vi "Autonomous Independent.vi"   [LabVIEW 2011]
doc: "This VI is called when autonomous begins, and will automatically be terminated when autonomous ends. You can carry out timed or sensor driven robot movement independently without needing to return to the caller."
uses:
  Robot Global Data.vi
  <vilib>/Rock Robotics/WPI/RobotDrive/WPI_RobotDriveArcadeDrive_Standard(NoSaturation).vi
types:
  T1 = typedef "WPI_RobotDriveDevRef.ctl" = cluster{"DevStatus":errorcluster, "Motors[]":T2[], "Square Inputs":bool, "Max Output":dbl, "Isochronous":bool}
  T2 = typedef "WPI_MotorControlDeviceRef.ctl" = cluster{"DeviceStatus":errorcluster, "Type":enum16{"PWM", "CAN"}, "PWM":cluster{"Digital Module":T3, "PWM Channel":T4, "DeadBand":T5}, "CAN":cluster{"Device Number":u8, "Control Mode":T6, "Semaphore":T7, "Max Vout":dbl}, "Invert":bool, "TransformRef":T8, "InvTransformRef":T8}
  T3 = typedef "FPGA_TypedefDigitalModule.ctl" = enum16{"Digital Module 1", "Digital Module 2"}
  T4 = typedef "FPGA_DIOPWMChannel.ctl" = enum8{"PWM 1", "PWM 2", "PWM 3", "PWM 4", "PWM 5", "PWM 6", "PWM 7", "PWM 8", "PWM 9", "PWM 10", "Invalid"}
  T5 = typedef "WPI_PWMDeadband.ctl" = cluster{"Name":string, "maxPositivePwm":i32, "minPositivePwm":i32, "centerPwm":i32, "maxNegativePwm":i32, "minNegativePwm":i32, "angularRange":u16}
  T6 = typedef "WPI_CANJaguar_ControlMode.ctl" = enum8{"Percent VBus", "Current", "Speed", "Position", "Voltage"}
  T7 = typedef "Semaphore RefNum" = refnum<k1>
  T8 = typedef "WPI_PWMTransform_ConPane.ctl" = refnum<vi>
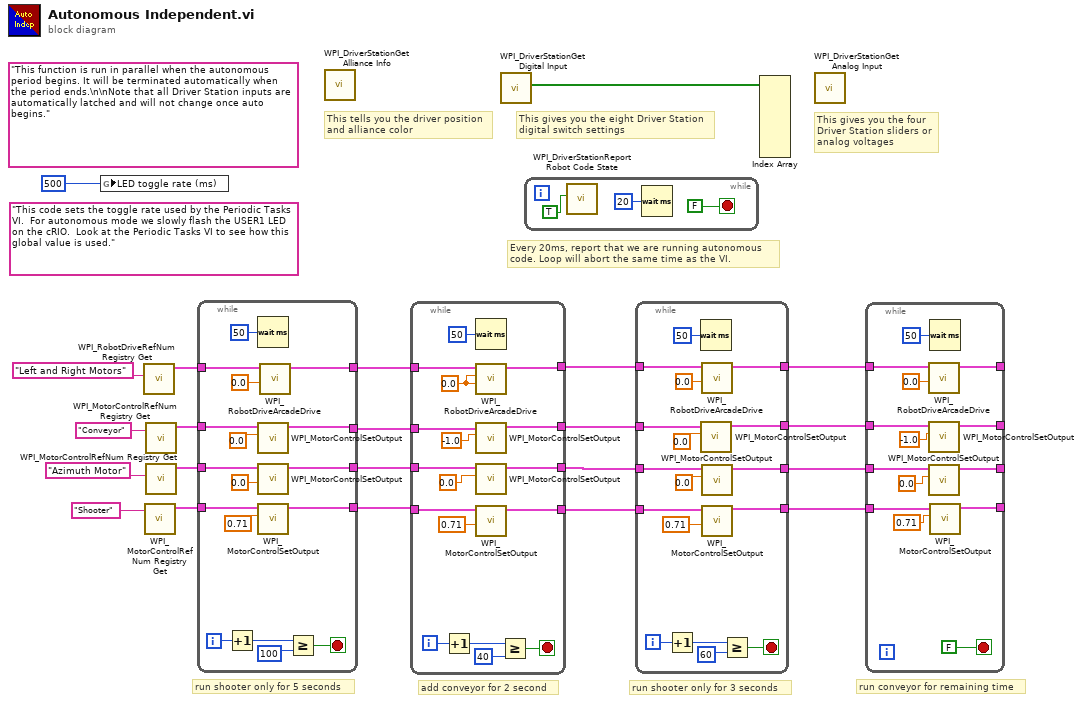
[diagram p0: block diagram]
diagram:
  (unwired) "This code sets the toggle rate used by the Periodic Tasks VI.  For autonomous mode we slowly flash the USER1 LED on the cRIO.  Look at the Periodic Tasks VI to see how this global value is used."
  (unwired) "This function is run in parallel when the autonomous period begins. It will be terminated automatically when the period ends.\n\nNote that all Driver Station inputs are automatically latched and will not change once auto begins."
  # "run conveyor for remaining time"
  # "run shooter only for 3 seconds"
  # "add conveyor for 2 second"
  # "run shooter only for 5 seconds"
  # "Every 20ms, report that we are running autonomous\ncode. Loop will abort the same time as the VI."
  # "This tells you the driver position\nand alliance color"
  # "This gives you the eight Driver Station\ndigital switch settings"
  # "This gives you the four\nDriver Station sliders or\nanalog voltages"
  n1 = global write "Robot Global Data.vi" "LED toggle rate (ms)"(u32 500 ("LED ms toggle rate")) -> ()
  n2 = call <vilib>:"WPI_RobotDriveRefNum Registry Get.vi"("refnum name"="Left and Right Motors") -> ("RobotDriveDevRef"=w8:T1)  [unwired: 9 in, 1 out]
  n3 = call <vilib>:"WPI_MotorControlRefNum Registry Get.vi"("refnum name"="Shooter") -> ("MotorControlDevRef"=w19:T2)  [unwired: 9 in, 1 out]
  n4 = call <vilib>:"WPI_MotorControlRefNum Registry Get.vi"("refnum name"="Conveyor") -> ("MotorControlDevRef"=w17:T2)  [unwired: 9 in, 1 out]
  n5 = call <vilib>:"WPI_MotorControlRefNum Registry Get.vi"("refnum name"="Azimuth Motor") -> ("MotorControlDevRef"=w3:T2)  [unwired: 9 in, 1 out]
  n6 = while {
    tunnel: w19 -> [w33]
    tunnel: [w34] -> w15
    tunnel: w17 -> [w32]
    tunnel: [w29] -> w16
    tunnel: w8 -> [w28]
    tunnel: [w27] -> w7
    tunnel: [w25] -> w4
    tunnel: w3 -> [w24]
    i -> [w38]
    stop <- w36 stop-if-true
    w23 = 0.0 ("Y axis value")
    n7 = Increment(x=w38) -> (x+1=w35:i32)
    n8 = Wait (ms)(milliseconds to wait=u32 50) -> ()  [unwired: 1 out]
    n9 = call <vilib>:"WPI_MotorControlSetOutput.vi"("Output"=0.0, "MotorControlDevRef"=w32) -> ("MotorControlDevRef"=w29:T2)  [unwired: 8 in, 1 out]
    n10 = call <vilib>:"WPI_MotorControlSetOutput.vi"("Output"=0.0, "MotorControlDevRef"=w24) -> ("MotorControlDevRef"=w25:T2)  [unwired: 8 in, 1 out]
    n11 = call <vilib>:"WPI_MotorControlSetOutput.vi"("Output"=0.71, "MotorControlDevRef"=w33) -> ("MotorControlDevRef"=w34:T2)  [unwired: 8 in, 1 out]
    n12 = call-poly <vilib>:"WPI_RobotDriveArcadeDrive.vi"("Y axis value"=w23, "X axis value"=w23, "RobotDriveDevRef"=w28) -> ("RobotDriveDevRef"=w27:T1)  [unwired: 7 in, 1 out]
    n13 = Greater Or Equal?(x=w35, y=100) -> (x >= y?=w36:bool)
  }
  n14 = call <vilib>:"WPI_DriverStationGet Alliance Info.vi"() -> ()  [unwired: 12 out]
  n15 = while {
    tunnel: w16 -> [w51]
    tunnel: w15 -> [w49]
    tunnel: [w47] -> w14
    tunnel: [w46] -> w13
    tunnel: w7 -> [w45]
    tunnel: [w44] -> w6
    tunnel: w4 -> [w42]
    tunnel: [w41] -> w2
    i -> [w55]
    stop <- w53 stop-if-true
    w40 = 0.0 ("X axis value")
    n16 = Increment(x=w55) -> (x+1=w52:i32)
    n17 = Wait (ms)(milliseconds to wait=u32 50) -> ()  [unwired: 1 out]
    n18 = call-poly <vilib>:"WPI_RobotDriveArcadeDrive.vi"("Y axis value"=w40, "X axis value"=w40, "RobotDriveDevRef"=w45) -> ("RobotDriveDevRef"=w44:T1)  [unwired: 7 in, 1 out]
    n19 = call <vilib>:"WPI_MotorControlSetOutput.vi"("Output"=-1.0, "MotorControlDevRef"=w51) -> ("MotorControlDevRef"=w46:T2)  [unwired: 8 in, 1 out]
    n20 = call <vilib>:"WPI_MotorControlSetOutput.vi"("Output"=0.0, "MotorControlDevRef"=w42) -> ("MotorControlDevRef"=w41:T2)  [unwired: 8 in, 1 out]
    n21 = call <vilib>:"WPI_MotorControlSetOutput.vi"("Output"=0.71, "MotorControlDevRef"=w49) -> ("MotorControlDevRef"=w47:T2)  [unwired: 8 in, 1 out]
    n22 = Greater Or Equal?(x=w52, y=40) -> (x >= y?=w53:bool)
  }
  n23 = call <vilib>:"WPI_DriverStationGet Digital Input.vi"() -> ("Driver Station Digital Input (1-8)"=w22:bool[])  [unwired: 11 out]
  n24 = while {
    stop <- FALSE stop-if-true
    n25 = call <vilib>:"WPI_DriverStationReport Robot Code State.vi"("Autonomous"=TRUE) -> ()  [unwired: 10 in, 1 out]
    n26 = Wait (ms)(milliseconds to wait=u32 20) -> ()  [unwired: 1 out]
  }
  n27 = while {
    tunnel: w14 -> [w75]
    tunnel: w13 -> [w74]
    tunnel: [w67] -> w12
    tunnel: [w66] -> w11
    tunnel: w6 -> [w65]
    tunnel: [w64] -> w5
    tunnel: w2 -> [w62]
    tunnel: [w61] -> w1
    i -> [w69]
    stop <- w68 stop-if-true
    w60 = 0.0 ("X axis value")
    n28 = Increment(x=w69) -> (x+1=w70:i32)
    n29 = Wait (ms)(milliseconds to wait=u32 50) -> ()  [unwired: 1 out]
    n30 = call <vilib>:"WPI_MotorControlSetOutput.vi"("Output"=0.0, "MotorControlDevRef"=w74) -> ("MotorControlDevRef"=w66:T2)  [unwired: 8 in, 1 out]
    n31 = call-poly <vilib>:"WPI_RobotDriveArcadeDrive.vi"("Y axis value"=w60, "X axis value"=w60, "RobotDriveDevRef"=w65) -> ("RobotDriveDevRef"=w64:T1)  [unwired: 7 in, 1 out]
    n32 = call <vilib>:"WPI_MotorControlSetOutput.vi"("Output"=0.0, "MotorControlDevRef"=w62) -> ("MotorControlDevRef"=w61:T2)  [unwired: 8 in, 1 out]
    n33 = call <vilib>:"WPI_MotorControlSetOutput.vi"("Output"=0.71, "MotorControlDevRef"=w75) -> ("MotorControlDevRef"=w67:T2)  [unwired: 8 in, 1 out]
    n34 = Greater Or Equal?(x=w70, y=60) -> (x >= y?=w68:bool)
  }
  n35 = Index Array(array=w22) -> ()  [unwired: 8 in, 8 out]
  n36 = call <vilib>:"WPI_DriverStationGet Analog Input.vi"() -> ()  [unwired: 12 out]
  n37 = while {
    tunnel: w11 -> [w89]
    tunnel: w12 -> [w86]
    tunnel: [w84] -> _
    tunnel: [w83] -> _
    tunnel: w5 -> [w82]
    tunnel: [w81] -> _
    tunnel: w1 -> [w79]
    tunnel: [w77] -> _
    stop <- FALSE stop-if-true
    w78 = 0.0 ("Y axis value")
    n38 = call-poly <vilib>:"WPI_RobotDriveArcadeDrive.vi"("Y axis value"=w78, "X axis value"=w78, "RobotDriveDevRef"=w82) -> ("RobotDriveDevRef"=w81:T1)  [unwired: 7 in, 1 out]
    n39 = call <vilib>:"WPI_MotorControlSetOutput.vi"("Output"=-1.0, "MotorControlDevRef"=w89) -> ("MotorControlDevRef"=w83:T2)  [unwired: 8 in, 1 out]
    n40 = call <vilib>:"WPI_MotorControlSetOutput.vi"("Output"=0.0, "MotorControlDevRef"=w79) -> ("MotorControlDevRef"=w77:T2)  [unwired: 8 in, 1 out]
    n41 = Wait (ms)(milliseconds to wait=u32 50) -> ()  [unwired: 1 out]
    n42 = call <vilib>:"WPI_MotorControlSetOutput.vi"("Output"=0.71, "MotorControlDevRef"=w86) -> ("MotorControlDevRef"=w84:T2)  [unwired: 8 in, 1 out]
  }
